vi "read_data.vi"(11 "Data path":path) -> (0 "scores":dbl[](array[numeric]), 1 "n":dbl, 2 "bboxes":T1(array[cluster]), 3 "classes":string[](array[string]))   [LabVIEW 2024]
uses:
  <vilib>/Utility/file.llb/Read Delimited Spreadsheet (string).vi
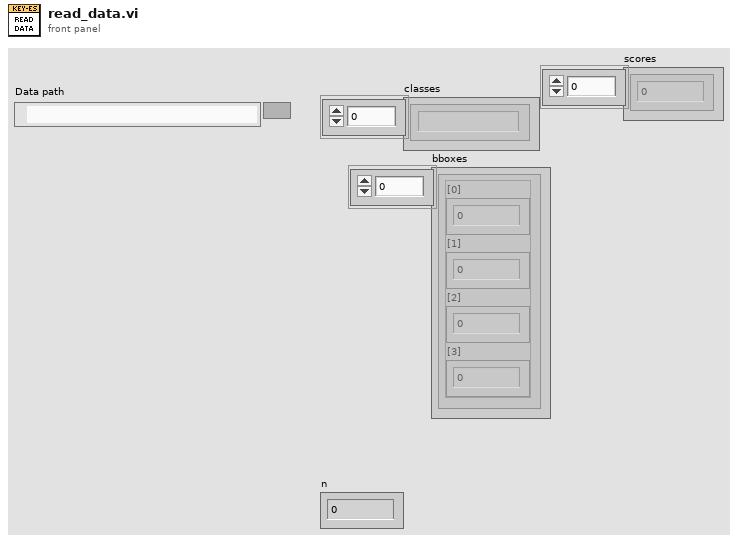
[diagram p1: front panel]
types:
  T1 = cluster{"[0]":dbl, "[1]":dbl, "[2]":dbl, "[3]":dbl}[]
  T2 = cluster{"[0]":i32, "[1]":i32, "[2]":i32, "[3]":i32}
  T3 = cluster{"[0]":dbl, "[1]":dbl, "[2]":dbl, "[3]":dbl}
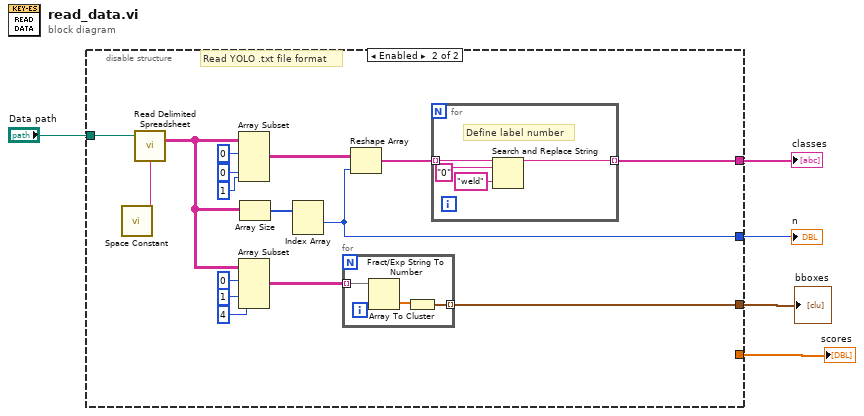
[diagram p0: block diagram]
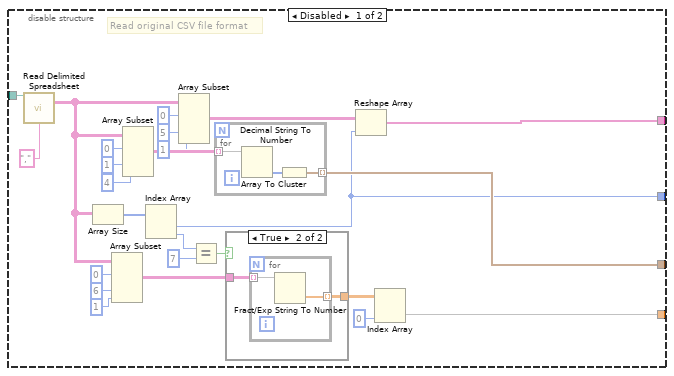
[diagram p2: hidden frame]
diagram:
  n1 = disable-structure shown="Enabled" {
    disable-tunnel: [w27 w38] -> w1
    disable-tunnel: "Data path" -> [w21 w53]
    disable-tunnel: [w19 w45] -> w4
    disable-tunnel: [w17 w44] -> w3
    disable-tunnel: [w6 _] -> w2
    frame Disabled {
      # "Read original CSV file format"
      n2 = call-poly <vilib>:"Read Delimited Spreadsheet.vi"("file path (dialog if empty)"=w21, "delimiter (\\t)"="," ("delimiter (\\t)")) -> ("all rows"=w16:string[][])  [unwired: 8 in, 5 out]
      n3 = Array Size(array=w16) -> (size(s)=w28:i32[])
      n4 = Array Subset(array=w16, index (row)=0 ("index"), index (col)=6 ("index"), length (col)=1 ("length")) -> (w9:string[][])  [unwired: 1 in]
      n5 = Array Subset(array=w16, index (row)=0 ("index"), index (col)=1 ("index"), length (col)=4 ("index")) -> (w26:string[][])  [unwired: 1 in]
      n6 = Index Array(array=w28) -> (element #1=w17:i32, element #2=w12:i32)  [unwired: 2 in]
      n7 = Array Subset(array=w16, index (row)=0 ("index"), index (col)=5 ("index"), length (col)=1 ("length")) -> (w20:string[][])  [unwired: 1 in]
      n8 = Equal?(x=w12, y=7) -> (x = y?=w10:bool)
      n9 = for {
        tunnel: w26 -> [w33] mode=indexing
        tunnel: [w31] -> w27 mode=indexing
        n10 = Decimal String To Number(string=w33) -> (number=w32:i32[])  [unwired: 2 in, 1 out]
        n11 = Array To Cluster(array=w32) -> (cluster=w31:T2)
      }
      n12 = case shown="True" w10 {
        tunnel: [_ w35] -> w7
        tunnel: w9 -> [_ w34]
        frame False {
        }
        frame True {
          n13 = for {
            tunnel: [w37] -> w35 mode=indexing
            tunnel: w34 -> [w36] mode=indexing
            n14 = Fract/Exp String To Number(string=w36) -> (number=w37:dbl[])  [unwired: 3 in, 1 out]
          }
        }
      }
      n15 = Reshape Array(w20, w17) -> (w19:string[])
      n16 = Index Array(array=w7, index (col)=0 ("disabled index (col)")) -> (element=w6:dbl[])  [unwired: 1 in]
    }
    frame Enabled {
      # "Read YOLO .txt file format"
      n17 = call <vilib>:"Space Constant.vi"() -> ("String"=w49:string)
      n18 = call-poly <vilib>:"Read Delimited Spreadsheet.vi"("file path (dialog if empty)"=w53, "delimiter (\\t)"=w49) -> ("all rows"=w40:string[][])  [unwired: 8 in, 5 out]
      n19 = Array Subset(array=w40, index (row)=0 ("index"), index (col)=0 ("index"), length (col)=1 ("length")) -> (w47:string[][])  [unwired: 1 in]
      n20 = Array Subset(array=w40, index (row)=0 ("index"), index (col)=1 ("index"), length (col)=4 ("index")) -> (w39:string[][])  [unwired: 1 in]
      n21 = Array Size(array=w40) -> (size(s)=w48:i32[])
      n22 = Index Array(array=w48) -> (element #1=w44:i32)  [unwired: 2 in, 1 out]
      n23 = for {
        tunnel: w39 -> [w56] mode=indexing
        tunnel: [w54] -> w38 mode=indexing
        n24 = Fract/Exp String To Number(string=w56) -> (number=w55:dbl[])  [unwired: 3 in, 1 out]
        n25 = Array To Cluster(array=w55) -> (cluster=w54:T3)
      }
      n26 = Reshape Array(w47, w44) -> (w46:string[])
      n27 = for {
        tunnel: w46 -> [w60] mode=indexing
        tunnel: [w57] -> w45 mode=indexing
        # "Define label number"
        n28 = Search and Replace String(input string=w60, search string="0", replace string="weld" ("replace string (\"\")")) -> (result string=w57:string)  [unwired: 5 in, 3 out]
      }
    }
  }
  "classes" <- w4
  "n" <- w3
  "scores" <- w2
  "bboxes" <- w1
